vi "Open Sensors.vi"   [LabVIEW 2016]
uses:
  Robot Global Data.vi
  <vilib>/Rock Robotics/WPI/Switch/WPI_SwitchOpenLimit.vi
  <vilib>/Rock Robotics/WPI/Counter/WPI_CounterDigitalInputToDigitalSource.vi
types:
  T1 = typedef "FPGA_DIOChannel.ctl" = enum8{"DIO 0", "DIO 1", "DIO 2", "DIO 3", "DIO 4", "DIO 5", "DIO 6", "DIO 7", "DIO 8", "DIO 9", "DIO MXP 0", "DIO MXP 1", "DIO MXP 2", "DIO MXP 3", "DIO MXP 4", "DIO MXP 5", "DIO MXP 6", "DIO MXP 7", "DIO MXP 8", "DIO MXP 9", "DIO MXP 10", "DIO MXP 11", "DIO MXP 12", "DIO MXP 13", "DIO MXP 14", "DIO MXP 15", "SPI Port CS1", "SPI Port CS2", "SPI Port CS3", "SPI Port MISO", "SPI Port MOSI", "Invalid"}
  T2 = cluster{"Lift Motors":cluster{"Left Lift":dbl, "Right Lift":dbl}, "Sensors":cluster{"Limit Switches":cluster{"Top IR":T1, "Bottom IR":T1, "Lift Safety":T1}, "Encoders":cluster{"Lift Encoder A Pin":T1, "Lift Encoder B Pin":T1}}, "Solenoids":cluster{"Left Clamp FWD":dbl, "Right Clamp FWD":dbl, "Brake BCK":dbl, "Left Clamp BCK":dbl, "Right Clamp BCK":dbl, "Left Clamp PModule":dbl, "Right Clamp PModule":dbl, "Brake PModule":dbl, "Brake FWD":dbl}, "Drive Motors":cluster{"Rear Left Motor":dbl, "Rear Right Motor":dbl, "Front Left Motor":dbl, "Front Right Motor":dbl}}
  T3 = typedef "WPI_DigitalInputDevRef.ctl" = cluster{"DevStatus":errorcluster, "DIO Channel":T1}
  T4 = typedef "WPI_SwitchDevRef.ctl" = cluster{"DevStatus":errorcluster, "DIO Channel":T1, "CntIndex":T5, "Normally Closed":bool}
  T5 = typedef "FPGA_CounterCtrSystemIndex.ctl" = enum8{"Ctr 0", "Ctr 1", "Ctr 2", "Ctr 3", "Ctr 4", "Ctr 5", "Ctr 6", "Ctr 7", "Invalid"}
  T6 = typedef "FPGA_CounterEncoderSourceConvertionLVSourceType.ctl" = cluster{"DevStatus":errorcluster, "AnalogTriggerMode?":bool, "DigitalMode":cluster{"DIO Channel":T7}, "AnalogTriggerMode":cluster{"AnalogTriggerIndex":T8, "OutputType":T9}}
  T7 = typedef "FPGA_DIODigitalSourceChannel.ctl" = enum8{"DIO 0", "DIO 1", "DIO 2", "DIO 3", "DIO 4", "DIO 5", "DIO 6", "DIO 7", "DIO 8", "DIO 9", "DIO MXP 0", "DIO MXP 1", "DIO MXP 2", "DIO MXP 3", "DIO MXP 4", "DIO MXP 5", "DIO MXP 6", "DIO MXP 7", "DIO MXP 8", "DIO MXP 9", "DIO MXP 10", "DIO MXP 11", "DIO MXP 12", "DIO MXP 13", "DIO MXP 14", "DIO MXP 15", "Disabled"}
  T8 = typedef "FPGA_AnalogTriggerIndex.ctl" = enum8{"Trig 0", "Trig 1", "Trig 2", "Trig 3", "Trig 4", "Trig 5", "Trig 6", "Trig 7", "Invalid"}
  T9 = typedef "FPGA_AnalogTriggerOutType.ctl" = enum16{"InWindow", "TriggerState", "Rising", "Falling"}
  T10 = typedef "WPI_EncoderDevRef.ctl" = cluster{"DevStatus":errorcluster, "EncoderIndex":T11, "CounterIndex":T5, "DistancePerCount":dbl, "Decoding Type":T12}
  T11 = typedef "FPGA_EncoderIdx.ctl" = enum8{"Enc 0", "Enc 1", "Enc 2", "Enc 3", "Enc 4", "Enc 5", "Enc 6", "Enc 7", "Invalid"}
  T12 = typedef "WPI_EncoderType.ctl" = enum16{"1x", "2x", "4x"}
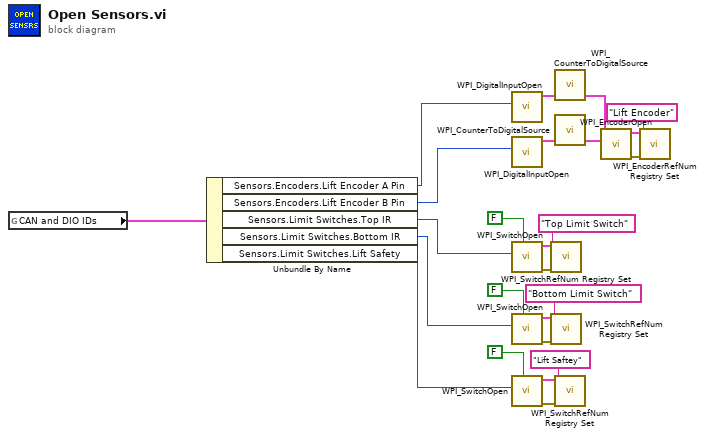
[diagram p0: block diagram]
diagram:
  n1 = global read "Robot Global Data.vi" "CAN and DIO IDs"() -> (w21:T2)
  n2 = Unbundle By Name(w21) -> ("Sensors.Encoders.Lift Encoder A Pin"=w20:T1, "Sensors.Encoders.Lift Encoder B Pin"=w19:T1, "Sensors.Limit Switches.Top IR"=w7:T1, "Sensors.Limit Switches.Bottom IR"=w6:T1, "Sensors.Limit Switches.Lift Safety"=w4:T1)
  n3 = call <vilib>:"WPI_DigitalInputOpen.vi"("DIO Channel"=w20) -> ("DigitalInputDevRef"=w23:T3)  [unwired: 1 in, 9 out]
  n4 = call <vilib>:"WPI_DigitalInputOpen.vi"("DIO Channel"=w19) -> ("DigitalInputDevRef"=w24:T3)  [unwired: 1 in, 9 out]
  n5 = call-poly <vilib>:"WPI_SwitchOpen.vi"("Normally Closed"=FALSE, "DIO Channel"=w7) -> ("error out"=w11:errorcluster, "SwitchDevRef"=w10:T4)  [unwired: 8 in]
  n6 = call-poly <vilib>:"WPI_SwitchOpen.vi"("Normally Closed"=FALSE, "DIO Channel"=w6) -> ("error out"=w13:errorcluster, "SwitchDevRef"=w12:T4)  [unwired: 8 in]
  n7 = call-poly <vilib>:"WPI_SwitchOpen.vi"("Normally Closed"=FALSE, "DIO Channel"=w4) -> ("error out"=w3:errorcluster, "SwitchDevRef"=w2:T4)  [unwired: 8 in]
  n8 = call <vilib>:"WPI_SwitchRefNum Registry Set.vi"("error in (no error)"=w11, "refnum name"="Top Limit Switch", "SwitchDevRef"=w10) -> ()  [unwired: 7 in, 2 out]
  n9 = call <vilib>:"WPI_SwitchRefNum Registry Set.vi"("error in (no error)"=w13, "refnum name"="Bottom Limit Switch", "SwitchDevRef"=w12) -> ()  [unwired: 7 in, 2 out]
  n10 = call-poly <vilib>:"WPI_CounterToDigitalSource.vi"("DigitalInputDevRef"=w23) -> ("Digital Source"=w22:T6)  [unwired: 6 out]
  n11 = call-poly <vilib>:"WPI_CounterToDigitalSource.vi"("DigitalInputDevRef"=w24) -> ("Digital Source"=w25:T6)  [unwired: 6 out]
  n12 = call <vilib>:"WPI_SwitchRefNum Registry Set.vi"("error in (no error)"=w3, "refnum name"="Lift Saftey", "SwitchDevRef"=w2) -> ()  [unwired: 7 in, 2 out]
  n13 = call <vilib>:"WPI_EncoderOpen.vi"("BSource"=w25, "ASource"=w22) -> ("error out"=w18:errorcluster, "EncoderDevRef"=w17:T10)  [unwired: 6 in, 2 out]
  n14 = call <vilib>:"WPI_EncoderRefNum Registry Set.vi"("error in (no error)"=w18, "refnum name"="Lift Encoder", "EncoderDevRef"=w17) -> ()  [unwired: 7 in, 2 out]
